vi "Main.vi"(10 "Sub Panel":refnum<vi>, 11 "Module Admin":refnum<class "Delacor_lib_QMH_Module Admin.lvclass">) -> ()   [LabVIEW 2020, in "Analisis.lvlib"]
doc: "This template is based off of the Queued Message Handler design pattern and the Queued Message Handler project template that ships with LabVIEW.\n\nThe main difference is that the queue is private to this module and communication between modules is performed via Broadcast and Request events.\n\nRequest events are wrapped in public API methods and are handled in the Event Handling Loop (EHL) of this VI. Any module can register for Broadcast events sent by this module. The EHL generates messages based on user interface actions.\n\nThe Message Handling Loop (MHL) processes messages generated by the EHL, or by other messages. The messages are string values, so new messages can be added easily to the Message Cases case structure in the MHL. Each message cluster can also provide an optional value for Message Data, which is a variant that can be converted to whatever message-specific data is required.\n_____\nBased on Delacor QMH Project Template 5.0.0.82."
uses:
  Analisis.lvlib
  <vilib>/Delacor/Delacor QMH/Libraries/Module Admin_class/Delacor_lib_QMH_Module Admin.lvclass
  Module Data--cluster.ctl
  <vilib>/vision/Image Controls.llb/IMAQ Image.ctl
  Stop Argument--cluster.ctl
  <vilib>/Delacor/Delacor QMH/Libraries/Message Queue_class/Delacor_lib_QMH_Message Queue.lvclass/Delacor_lib_QMH_Message Queue.ctl
  <vilib>/Delacor/Delacor QMH/Libraries/Module Admin_class/Delacor_lib_QMH_Module Admin.lvclass/Delacor_lib_QMH_Module Admin.ctl
  <vilib>/Delacor/Delacor QMH/Libraries/Message Queue_class/Delacor_lib_QMH_Enqueue Message (Single).vi
  <vilib>/Delacor/Delacor QMH/Libraries/Module Admin_class/Delacor_lib_QMH_Get External Launch.vi
  <vilib>/Utility/error.llb/Error Cluster From Error Code.vi
  <vilib>/ErrorRing/Error Ring.xnode
  <vilib>/Delacor/Delacor QMH/Libraries/Message Queue_class/Delacor_lib_QMH_Message Queue.lvclass
  Database/Database.lvlib
panel:
  out "Color:":string
  out "Image":T1(plugin-control)
  out "Codigo:":string
  out "Usuario:":string
  out "Letra:":string
  out "error out":errorcluster
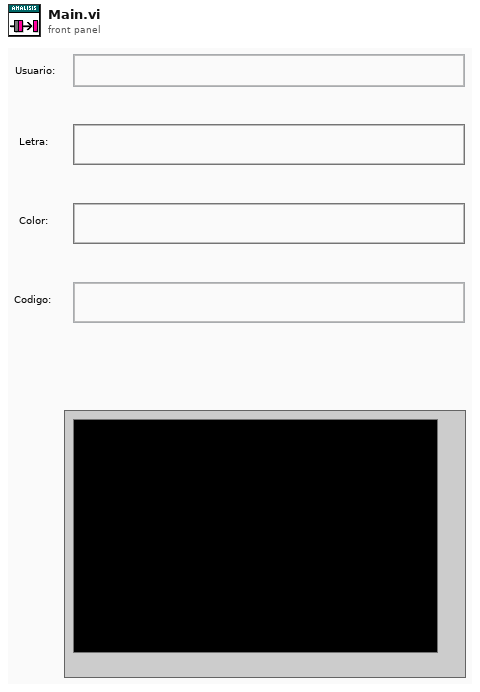
[diagram p1: front panel]
types:
  T1 = typedef "IMAQ Image.ctl" = refnum<image>
  T2 = typedef "Analisis.lvlib/Request Events--cluster.ctl" = cluster{"Stop Module":refnum<user-event>, "Show Panel":refnum<user-event>, "Hide Panel":refnum<user-event>, "Get Module Execution Status":refnum<user-event>, "Show Diagram":refnum<user-event>, "Start":refnum<user-event>, "stop analisis":refnum<user-event>}
  T3 = typedef "Analisis.lvlib/Module Data--cluster.ctl" = cluster{"Image Src":T1}
  T4 = enum32{"Invalid", "Standard", "Closed", "Hidden", "Minimized", "Maximized"}
  T5 = typedef "Analisis.lvlib/Stop Argument--cluster.ctl" = cluster{"Origin":string, "Exit via Stop Module Req?":bool, "Wait for Module to stop?":bool}
  T6 = enum32{"invalid lock state", "Not Locked", "Locked (No Password)", "Password-protected"}
  T7 = cluster{"Classes (Color Classification 1)[0]":string, "Classes (Color Classification 1)[1]":string, "Classes (Color Classification 1)[2]":string, "Classes (Color Classification 1)[3]":string, "Classes (Color Classification 1)[4]":string, "Classes (Color Classification 1)[5]":string, "Classes (Color Classification 1)[6]":string, "Classes (Color Classification 1)[7]":string, "Classes (Color Classification 1)[8]":string}
  T8 = cluster{"Complete Data (Barcode Reader 1)[0]":string, "Complete Data (Barcode Reader 1)[1]":string, "Complete Data (Barcode Reader 1)[2]":string, "Complete Data (Barcode Reader 1)[3]":string, "Complete Data (Barcode Reader 1)[4]":string, "Complete Data (Barcode Reader 1)[5]":string, "Complete Data (Barcode Reader 1)[6]":string, "Complete Data (Barcode Reader 1)[7]":string, "Complete Data (Barcode Reader 1)[8]":string}
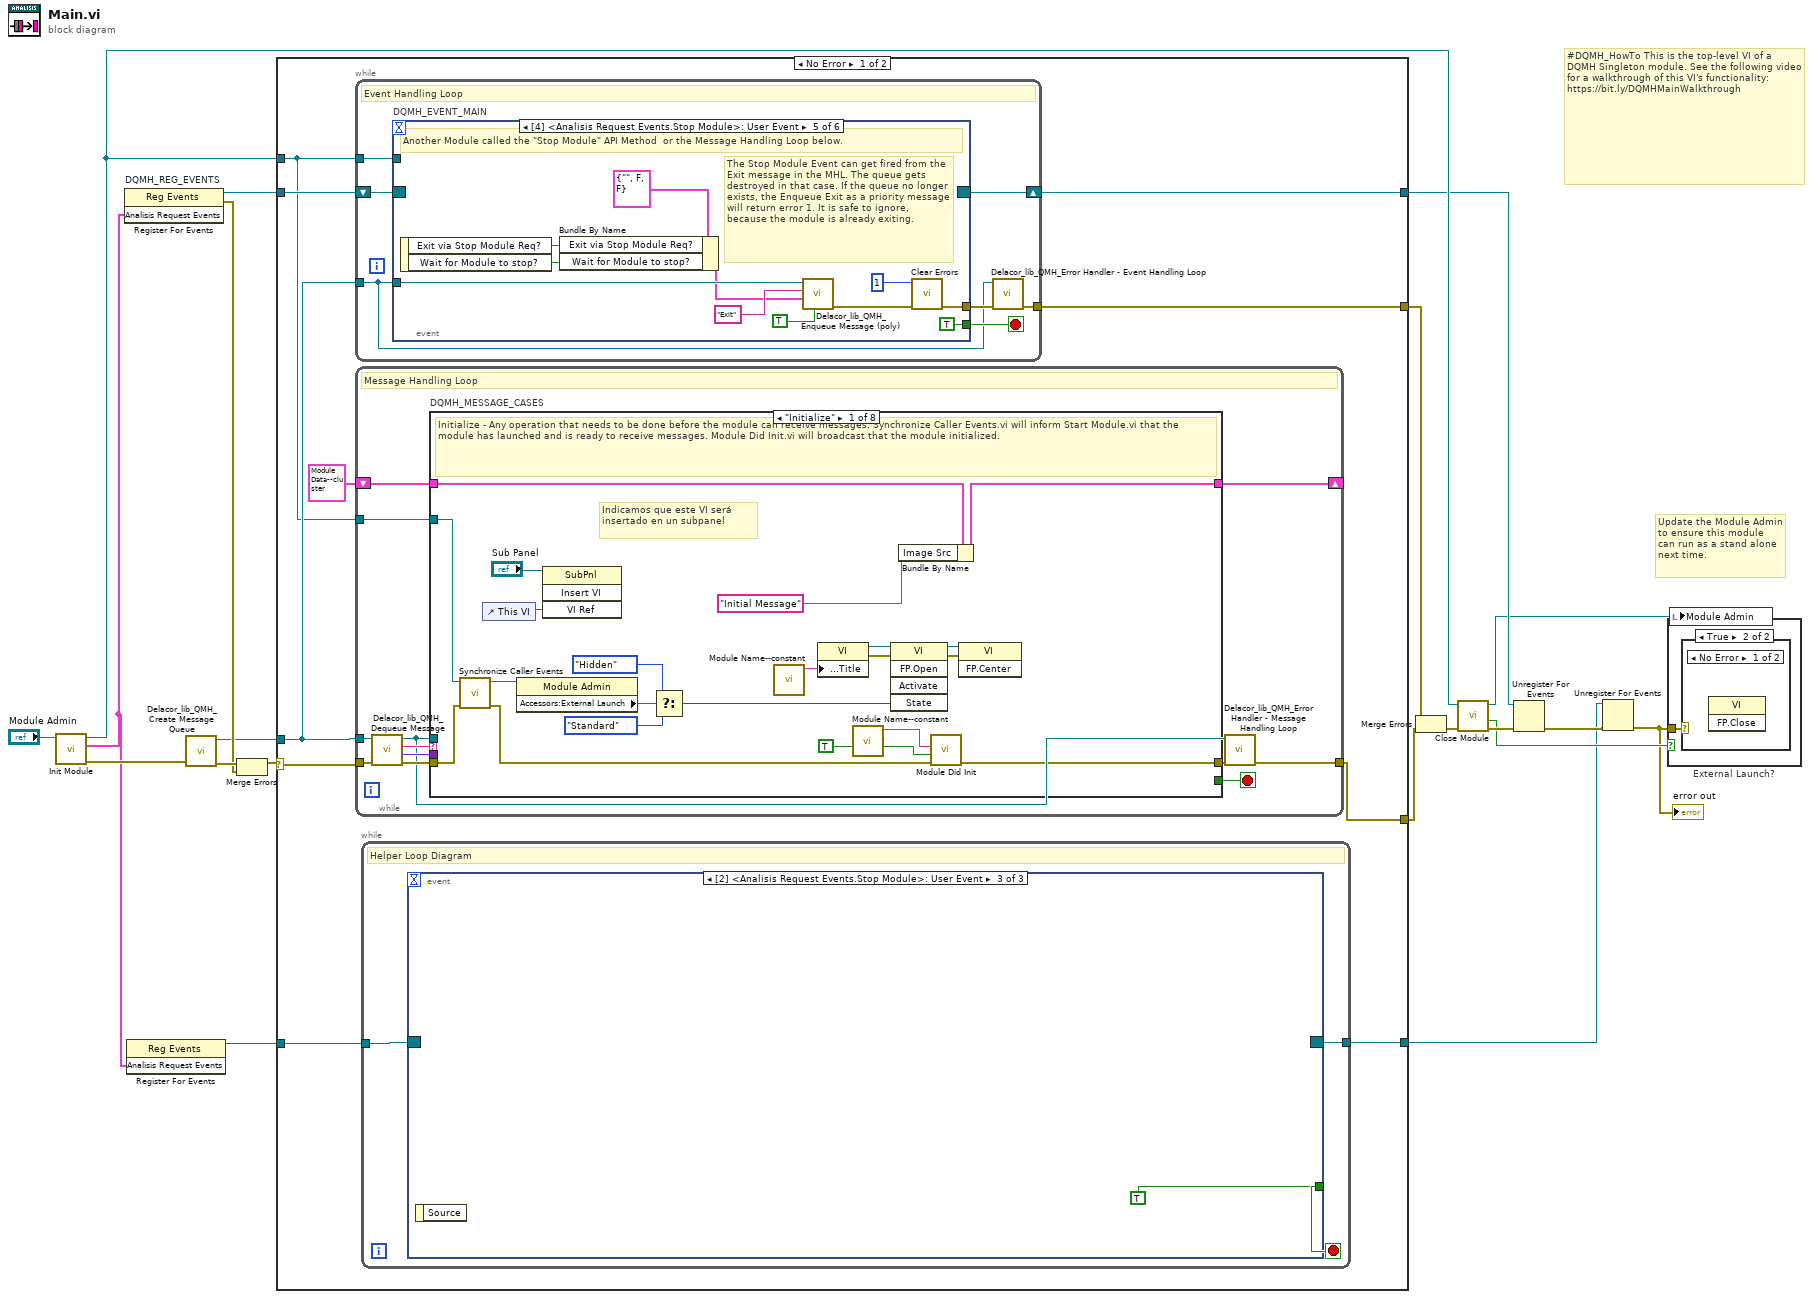
[diagram p0: block diagram]
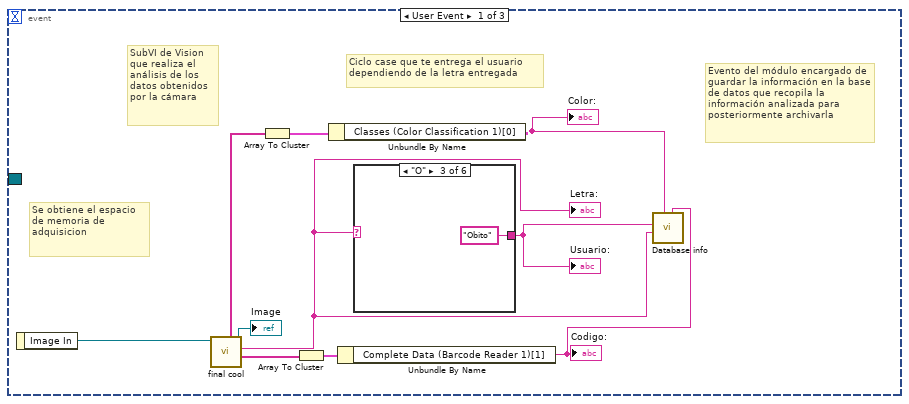
[diagram p2: hidden frame]
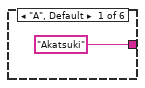
[diagram p3: hidden frame]
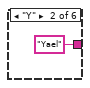
[diagram p4: hidden frame]
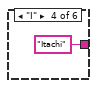
[diagram p5: hidden frame]
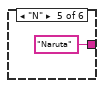
[diagram p6: hidden frame]
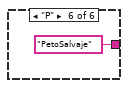
[diagram p7: hidden frame]
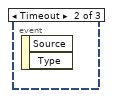
[diagram p8: hidden frame]
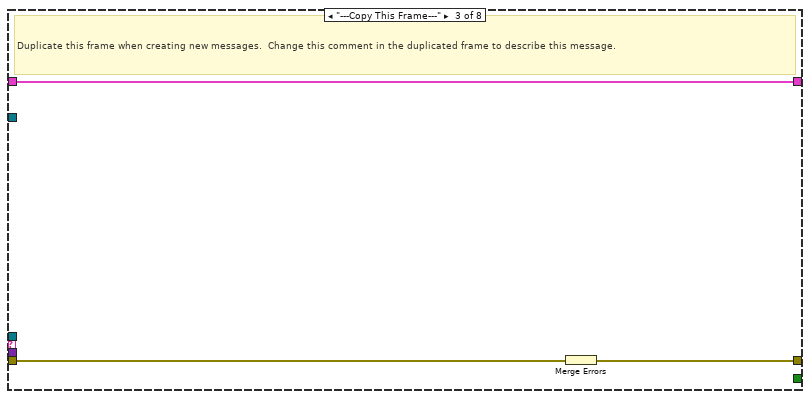
[diagram p10: hidden frame]
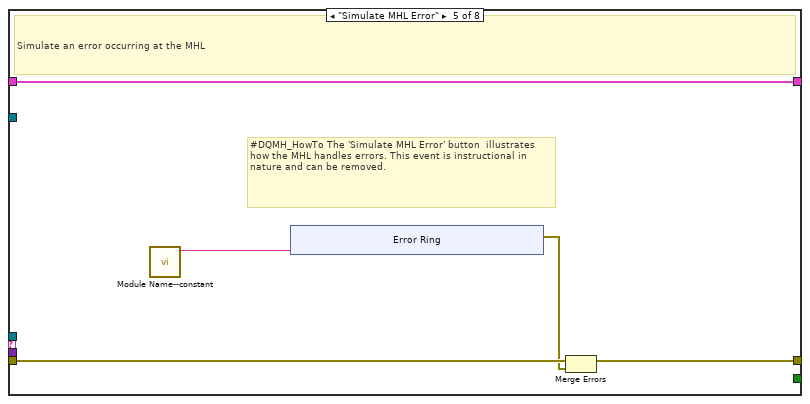
[diagram p12: hidden frame]
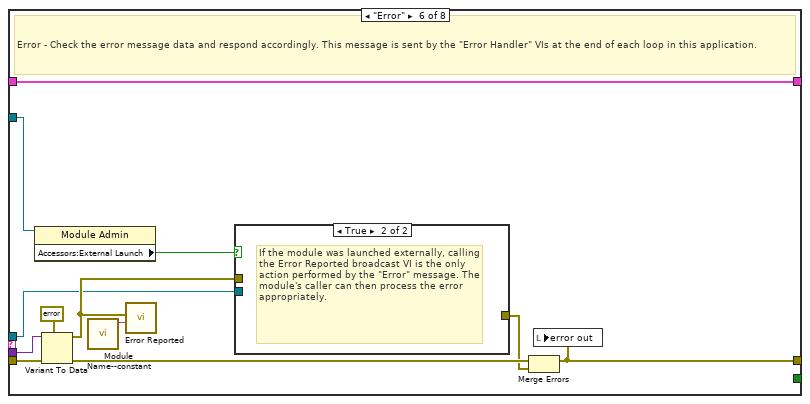
[diagram p13: hidden frame]
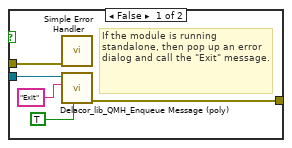
[diagram p14: hidden frame]
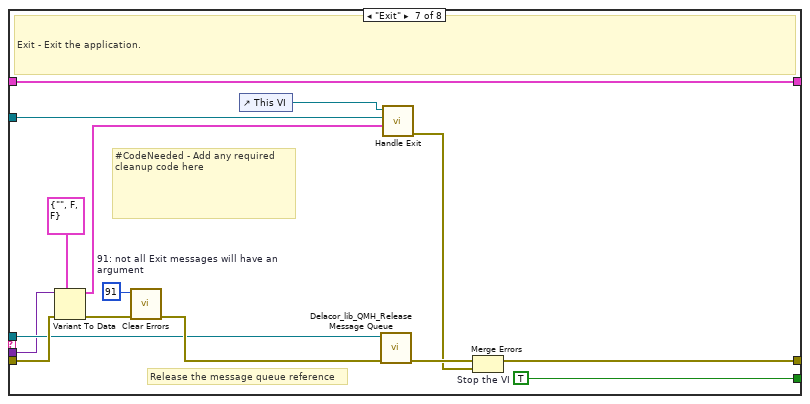
[diagram p15: hidden frame]
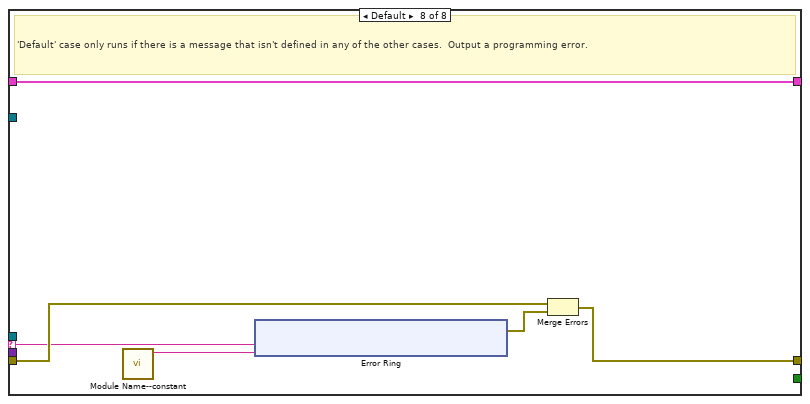
[diagram p16: hidden frame]
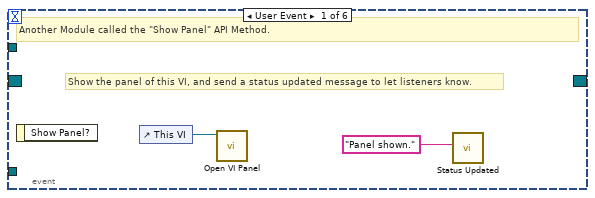
[diagram p17: hidden frame]
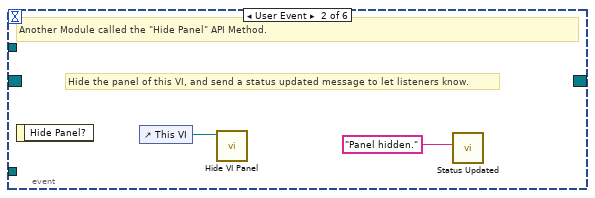
[diagram p18: hidden frame]
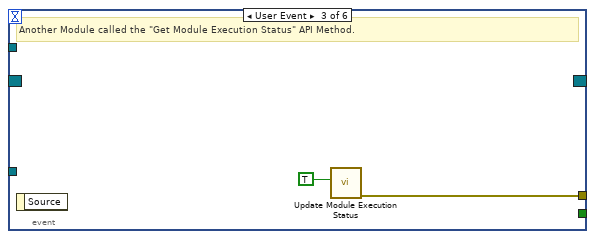
[diagram p19: hidden frame]
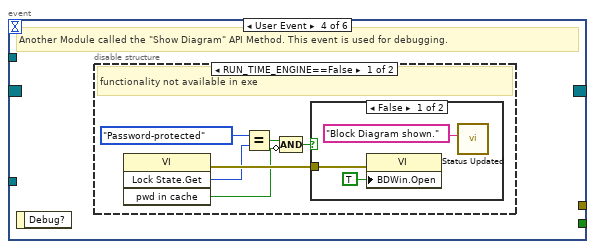
[diagram p20: hidden frame]
diagram:
  # "#DQMH_HowTo This is the top-level VI of a DQMH Singleton module. See the following video for a walkthrough of this VI's functionality: https://bit.ly/DQMHMainWalkthrough"
  # "Update the Module Admin to ensure this module can run as a stand alone next time."
  n1 = call "Init Module.vi"("Singleton Module Admin in"="Module Admin") -> ("error out"=w19:errorcluster, "Analisis Request Events"=w5:T2, "Singleton Module Admin out"=w12:refnum<class "Delacor_lib_QMH_Module Admin.lvclass">)  [unwired: 8 in]
  n2 = register-events "DQMH_REG_EVENTS"(w5) -> (reference out=w10:refnum<event-registration>, error out=w13:errorcluster)  [unwired: 2 in]
  n3 = register-events(w5) -> (reference out=w4:refnum<event-registration>)  [unwired: 2 in, 1 out]
  n4 = call <vilib>:"Delacor_lib_QMH_Create Message Queue.vi"("error in (no error)"=w19) -> ("error out"=w15:errorcluster, "Message Queue"=w9:refnum<class "Delacor_lib_QMH_Message Queue.lvclass">)  [unwired: 9 in]
  n5 = Merge Errors(w15, w13) -> (w14:errorcluster)
  n6 = case shown="No Error" w14 {
    selector: w14 -> [w28 w195]
    tunnel: [w30 w194] -> w20
    tunnel: [w27 w200] -> w11
    tunnel: w10 -> [w26 w200]
    tunnel: w9 -> [w25 w193]
    tunnel: [w29 _] -> w17
    tunnel: w12 -> [w24 w196]
    tunnel: w4 -> [w22 w192]
    tunnel: [w21 w192] -> w1
    frame No Error {
      n7 = while {
        tunnel: w25 -> [w149]
        shift-right: [w152] -> w27
        shift-left: w26 -> [w153]
        tunnel: [w154] -> w29
        tunnel: w24 -> [w150]
        stop <- w151 stop-if-true
        # "Event Handling Loop"
        n8 = event "DQMH_EVENT_MAIN" shown="[4] <Analisis Request Events.Stop Module>: User Event" {
          selector: w153 -> [_ _ _ _ _ _]
          dyn-events: [_ _ _ _ _ _] -> w152
          timeout: _ -> [_ _ _ _ _ _]
          tunnel: [_ _ _ _ TRUE ("Discard?") _] -> w151
          tunnel: w149 -> [_ _ _ _ w177 w184]
          tunnel: [_ _ w161 _ w180 w186] -> w155
          tunnel: w150 -> [_ _ _ _ _ w183]
          event User Event {
            # "Show the panel of this VI, and send a status updated message to let listeners know."
            # "Another Module called the \"Show Panel\" API Method."
            n9 = event-data() -> ()  [unwired: 1 in, 1 out]
            n10 = control-ref of="This VI"() -> (w157:refnum<vi>)
            n11 = call "Open VI Panel.vi"("VI"=w157) -> ()  [unwired: 10 in, 1 out]
            n12 = call "Status Updated.vi"("Status"="Panel shown." ("format string")) -> ()  [unwired: 10 in, 1 out]
          }
          event User Event {
            # "Hide the panel of this VI, and send a status updated message to let listeners know."
            # "Another Module called the \"Hide Panel\" API Method."
            n13 = event-data() -> ()  [unwired: 1 in, 1 out]
            n14 = control-ref of="This VI"() -> (w159:refnum<vi>)
            n15 = call "Hide VI Panel.vi"("VI"=w159) -> ()  [unwired: 10 in, 1 out]
            n16 = call "Status Updated.vi"("Status"="Panel hidden." ("format string")) -> ()  [unwired: 10 in, 1 out]
          }
          event User Event {
            # "Another Module called the \"Get Module Execution Status\" API Method."
            n17 = event-data() -> ()  [unwired: 1 in, 1 out]
            n18 = call "Update Module Execution Status.vi"("Running?"=TRUE) -> ("error out"=w161:errorcluster)  [unwired: 10 in]
          }
          event User Event {
            # "Another Module called the \"Show Diagram\" API Method. This event is used for debugging."
            n19 = event-data() -> ()  [unwired: 1 in, 1 out]
            n20 = disable-structure shown="RUN_TIME_ENGINE==False" {
              frame condition #0 (active) {
                # "functionality not available in exe"
                n21 = invoke class="VI" method="Lock State.Get"() -> (error out=w167:errorcluster, "Get Lock State"=w166:T6, "pwd in cache"=w163:bool)  [unwired: 4 in, 1 out]
                n22 = Equal?(x=T6."Password-protected", y=w166) -> (x = y?=w164:bool)
                n23 = Compound Arithmetic op=AND(w164, invert w163) -> (w162:bool)
                n24 = case shown="False" w162 {
                  tunnel: w167 -> [w170 _]
                  frame False {
                    n25 = property class="VI"(error in=w170, "BDWin.Open"=TRUE ("Block Diagram Window:Open")) -> ()  [unwired: 1 in, 2 out]
                    n26 = call "Status Updated.vi"("Status"="Block Diagram shown." ("format string")) -> ()  [unwired: 10 in, 1 out]
                  }
                  frame True {
                    # "Password-protected VI, and the password is not in the cache. Do not show the diagram."
                  }
                }
              }
              frame condition #1 {
              }
            }
          }
          event User Event {
            # "The Stop Module Event can get fired from the Exit message in the MHL. The queue gets destroyed in that case. If the queue no longer exists, the Enqueue Exit as a priority message will return error 1. It is safe to ignore, because the module is already exiting."
            # "Another Module called the \"Stop Module\" API Method  or the Message Handling Loop below."
            n27 = event-data() -> ("Exit via Stop Module Req?"=w173:bool, "Wait for Module to stop?"=w172:bool)  [unwired: 1 in]
            n28 = Bundle By Name(cluster=T5 {"Origin"="", "Exit via Stop Module Req?"=FALSE, "Wait for Module to stop?"=FALSE} ("Stop Argument"), "Exit via Stop Module Req?"=w173, "Wait for Module to stop?"=w172) -> (w171:T5)
            n29 = call-poly <vilib>:"Delacor_lib_QMH_Enqueue Message (poly).vi"("Priority Message? (F)"=TRUE, "Message Data"=w171, "Message"="Exit", "Message Queue in"=w177) -> ("error out"=w181:errorcluster)  [unwired: 6 in, 1 out]
            n30 = call <vilib>:"Clear Errors.vi"("error in (no error)"=w181, "specific error code to clear (0: all)"=1) -> ("error out"=w180:errorcluster)  [unwired: 4 in, 1 out]
          }
          event Panel Close? {
            w185 = TRUE  # Discard the event, the MHL is responsible for closing and stopping this VI.
            # "Hide the panel or send the 'Exit' message if the user clicks the 'X' on the module main VI panel."
            n31 = event-data() -> ()  [unwired: 1 in, 1 out]
            n32 = property class="Module Admin"(reference=w183) -> ("Accessors:External Launch"=w182:bool)  [unwired: 1 in, 2 out]
            n33 = case shown="True" w182 {
              tunnel: w184 -> [_ w190]
              tunnel: [_ w191] -> w186
              frame True {
                # "If externally launched, clicking the 'X' hides the panel, but doesn't close it."
                n34 = control-ref of="This VI"() -> (w187:refnum<vi>)
                n35 = call "Hide VI Panel.vi"("VI"=w187) -> ()  [unwired: 10 in, 1 out]
              }
              frame False {
                # "If run as a stand-alone VI, clicking the panel 'X' stops the VI."
                n36 = call-poly <vilib>:"Delacor_lib_QMH_Enqueue Message (poly).vi"("Priority Message? (F)"=TRUE, "Message"="Exit", "Message Queue in"=w190) -> ("error out"=w191:errorcluster)  [unwired: 7 in, 1 out]
              }
            }
            n37 = event-data("Discard?"=w185) -> ()  [unwired: 1 in, 1 out]
          }
        }
        n38 = call-dynamic "Delacor_lib_QMH_Error Handler - Event Handling Loop.vi"("error in (no error)"=w155, "Message Queue in"=w149) -> ("dup error in"=w154:errorcluster)  [unwired: 8 in, 1 out]
      }
      n39 = while {
        tunnel: w25 -> [w53]
        shift-right: [w57] -> _
        shift-left: T3 {"Image Src"=refnum} ("Data Cluster") -> [w58]
        tunnel: w28 -> [w61]
        tunnel: [w59] -> w30
        tunnel: w24 -> [w51]
        stop <- w56 stop-if-true
        # "Message Handling Loop"
        n40 = call-dynamic "Delacor_lib_QMH_Dequeue Message.vi"("error in (no error)"=w61, "Message Queue in"=w53) -> ("error out"=w60:errorcluster, "Message Data"=w54:variant, "Message"=w55:string, "Message Queue out"=w52:refnum<class "Delacor_lib_QMH_Message Queue.lvclass">)  [unwired: 6 in]
        n41 = case "DQMH_MESSAGE_CASES" shown="\"Initialize\"" w55 {
          selector: w55 -> [_ _ _ _ _ _ _ w136]
          tunnel: w52 -> [_ _ _ _ _ w106 w128 _]
          tunnel: w60 -> [w81 w85 w88 w90 w95 w113 w134 w138]
          tunnel: [w79 w85 w87 w90 w94 w109 w131 w139] -> w62
          tunnel: w58 -> [w70 w84 w86 w89 w92 w108 w127 w137]
          tunnel: [w69 w84 w86 w89 w92 w108 w127 w137] -> w57
          tunnel: [_ _ _ _ _ _ w126 _] -> w56
          tunnel: w54 -> [_ _ _ _ _ w107 w125 _]
          tunnel: w51 -> [w71 _ _ _ _ w105 w120 _]
          frame "Initialize" {
            # "Indicamos que este VI será insertado en un subpanel"
            # "Initialize - Any operation that needs to be done before the module can receive messages. Synchronize Caller Events.vi will inform Start Module.vi that the module has launched and is ready to receive messages. Module Did Init.vi will broadcast that the module initialized."
            n42 = call "Synchronize Caller Events.vi"("error in (no error)"=w81, "Singleton Module Admin in"=w71) -> ("error out"=w80:errorcluster, "Singleton Module Admin out"=w66:refnum<class "Delacor_lib_QMH_Module Admin.lvclass">)  [unwired: 8 in]
            n43 = control-ref of="This VI"() -> (w63:refnum<vi>)
            n44 = property class="Module Admin"(reference=w66) -> ("Accessors:External Launch"=w75:bool)  [unwired: 1 in, 2 out]
            n45 = invoke class="SubPnl" method="Insert VI"(reference="Sub Panel", "VI Ref"=w63) -> ()  [unwired: 2 in, 4 out]
            n46 = Select(t=T4."Hidden" ("State"), s=w75, f=T4."Standard" ("State")) -> (s? t:f=w72:T4)
            n47 = call "Module Name--constant.vi"() -> ("Module Name"=w78:string)  [unwired: 11 in]
            n48 = property class="VI"("Front Panel.Title"=w78) -> (reference out=w77:refnum<vi>, error out=w83:errorcluster)  [unwired: 2 in]
            n49 = call "Module Name--constant.vi"() -> ("Module Name"=w67:string)  [unwired: 11 in]
            n50 = invoke class="VI" method="FP.Open"(reference=w77, error in=w83, "State"=w72) -> (reference out=w76:refnum<vi>, error out=w82:errorcluster)  [unwired: 2 in, 3 out]
            n51 = Bundle By Name(cluster=w70, "Image Src"="Initial Message" ("Initial Message")) -> (w69:T3)
            n52 = call "Module Did Init.vi"("error in (no error)"=w80, "Initialized?"=TRUE, "Origin"=w67) -> ("error out"=w79:errorcluster)  [unwired: 8 in]
            n53 = invoke class="VI" method="FP.Center"(reference=w76, error in=w82) -> ()  [unwired: 1 in, 3 out]
          }
          frame "--- Module Specific ---" {
            # "Separator -- The following cases handle messages specific to this Module."
          }
          frame "---Copy This Frame---" {
            # "Duplicate this frame when creating new messages.  Change this comment in the duplicated frame to describe this message."
            n54 = Merge Errors(w88) -> (w87:errorcluster)
          }
          frame "--- Exit and Error Handling---" {
            # "Separator - The following cases handle errors and exit messages."
          }
          frame "Simulate MHL Error" {
            # "#DQMH_HowTo The 'Simulate MHL Error' button  illustrates how the MHL handles errors. This event is instructional in nature and can be removed."
            # "Simulate an error occurring at the MHL"
            n55 = call "Module Name--constant.vi"() -> ("Module Name"=w91:string)  [unwired: 11 in]
            n56 = xnode "Error Ring"("parameter 0"=w91) -> ("error out"=w93:errorcluster)
            n57 = Merge Errors(w95, w93) -> (w94:errorcluster)
          }
          frame "Error" {
            # "Error - Check the error message data and respond accordingly. This message is sent by the \"Error Handler\" VIs at the end of each loop in this application."
            n58 = property class="Module Admin"(reference=w105) -> ("Accessors:External Launch"=w104:bool)  [unwired: 1 in, 2 out]
            n59 = Variant To Data(error in=w113, type=errorcluster {"status"=FALSE, "code"=0, "source"=""} ("error constant"), Variant=w107) -> (data=w114:errorcluster, error out=w111:errorcluster)
            n60 = call "Module Name--constant.vi"() -> ("Module Name"=w103:string)  [unwired: 11 in]
            n61 = call "Error Reported.vi"("Additional Information"=w103, "Error"=w114) -> ()  [unwired: 9 in, 1 out]
            n62 = case shown="True" w104 {
              tunnel: [w119 _] -> w110
              tunnel: w106 -> [w117 _]
              tunnel: w114 -> [w118 _]
              frame False {
                # "If the module is running standalone, then pop up an error dialog and call the \"Exit\" message."
                n63 = call <vilib>:"Simple Error Handler.vi"("error in (no error)"=w118) -> ()  [unwired: 4 in, 5 out]
                n64 = call-poly <vilib>:"Delacor_lib_QMH_Enqueue Message (poly).vi"("Priority Message? (F)"=TRUE, "Message"="Exit", "Message Queue in"=w117) -> ("error out"=w119:errorcluster)  [unwired: 7 in, 1 out]
              }
              frame True {
                # "If the module was launched externally, calling the Error Reported broadcast VI is the only action performed by the \"Error\" message. The module's caller can then process the error appropriately."
              }
            }
            n65 = Merge Errors(w111, w110) -> (w109:errorcluster)
            n66 = local write "error out"(w109) -> ()
          }
          frame "Exit" {
            w124 = 91  # 91: not all Exit messages will have an argument
            w126 = TRUE  # Stop the VI
            # "Release the message queue reference"
            # "#CodeNeeded - Add any required cleanup code here"
            # "Exit - Exit the application."
            n67 = Variant To Data(error in=w134, type=T5 {"Origin"="", "Exit via Stop Module Req?"=FALSE, "Wait for Module to stop?"=FALSE} ("Stop Argument"), Variant=w125) -> (data=w122:T5, error out=w130:errorcluster)
            n68 = call <vilib>:"Clear Errors.vi"("error in (no error)"=w130, "specific error code to clear (0: all)"=w124) -> ("error out"=w133:errorcluster)  [unwired: 4 in, 1 out]
            n69 = control-ref of="This VI"() -> (w121:refnum<vi>)
            n70 = call-dynamic "Delacor_lib_QMH_Release Message Queue.vi"("error in (no error)"=w133, "Message Queue"=w128) -> ("error out"=w132:errorcluster)  [unwired: 9 in]
            n71 = call "Handle Exit.vi"("Stop Argument"=w122, "Admin in"=w120, "VI reference"=w121) -> ("error out"=w129:errorcluster)  [unwired: 7 in, 1 out]
            n72 = Merge Errors(w132, w129) -> (w131:errorcluster)
          }
          frame Default {
            # "'Default' case only runs if there is a message that isn't defined in any of the other cases.  Output a programming error."
            n73 = call "Module Name--constant.vi"() -> ("Module Name"=w135:string)  [unwired: 11 in]
            n74 = xnode "Error Ring"("parameter 0"=w136, "parameter 1"=w135) -> ("error out"=w140:errorcluster)
            n75 = Merge Errors(w138, w140) -> (w139:errorcluster)
          }
        }
        n76 = call-dynamic "Delacor_lib_QMH_Error Handler - Message Handling Loop.vi"("error in (no error)"=w62, "Message Queue in"=w52) -> ("dup error in"=w59:errorcluster)  [unwired: 8 in, 1 out]
      }
      n77 = while {
        tunnel: w22 -> [w33]
        tunnel: [w31] -> w21
        stop <- w32 stop-if-true
        # "Helper Loop Diagram"
        n78 = event shown="[2] <Analisis Request Events.Stop Module>: User Event" {
          selector: w33 -> [_ _ _]
          dyn-events: [_ _ _] -> w31
          timeout: _ -> [_ _ _]
          tunnel: [_ _ TRUE] -> w32
          event User Event {
            # "Ciclo case que te entrega el usuario dependiendo de la letra entregada"
            # "Evento del módulo encargado de guardar la información en la base de datos que recopila la información analizada para posteriormente archivarla"
            # "SubVI de Vision que realiza el análisis de los datos obtenidos por la cámara"
            # "Se obtiene el espacio de memoria de adquisicion"
            n79 = event-data() -> ("Image In"=w36:T1)  [unwired: 1 in]
            n80 = call "final cool.vi"("Image In"=w36) -> ("Complete Data (Barcode Reader 1)"=w38:string[], "String (OCR/OCV 1)"=w39:string, "Image Out"=→"Image":T1, "Classes (Color Classification 1)"=w40:string[])  [unwired: 6 in, 1 out]
            "Letra:" <- w39
            n81 = Array To Cluster(array=w40) -> (cluster=w42:T7)
            n82 = Array To Cluster(array=w38) -> (cluster=w37:T8)
            n83 = Unbundle By Name(w42) -> ("Classes (Color Classification 1)[0]"=w34:string)
            "Color:" <- w34
            n84 = Unbundle By Name(w37) -> ("Complete Data (Barcode Reader 1)[1]"=w35:string)
            "Codigo:" <- w35
            n85 = case shown="\"O\"" w39 {
              tunnel: ["Akatsuki" "Yael" "Obito" "Itachi" "Naruta" "PetoSalvaje"] -> w43
              frame "A", Default {
              }
              frame "Y" {
              }
              frame "O" {
              }
              frame "I" {
              }
              frame "N" {
              }
              frame "P" {
              }
            }
            "Usuario:" <- w43
            n86 = call "Database info.vi"("Codigo"=w35, "Color"=w34, "Letra"=w39, "usuario"=w43) -> ()  [unwired: 7 in, 1 out]
          }
          event Timeout {
            n87 = event-data() -> ()  [unwired: 1 in, 2 out]
          }
          event User Event {
            n88 = event-data() -> ()  [unwired: 1 in, 1 out]
          }
        }
      }
    }
    frame Error {
      # "Synchronize Caller Events.vi will inform Start Module.vi that the module has launched and will let the code calling Start Module.vi register for broadcasts and would permit the caller receive the broadcast that an error occurred at launch time."
      n89 = call-dynamic "Delacor_lib_QMH_Release Message Queue.vi"("error in (no error)"=w195, "Message Queue"=w193) -> ("error out"=w194:errorcluster)  [unwired: 9 in]
      n90 = call "Synchronize Caller Events.vi"("Singleton Module Admin in"=w196) -> ("error out"=w201:errorcluster)  [unwired: 9 in, 1 out]
      n91 = call "Module Name--constant.vi"() -> ("Module Name"=w199:string)  [unwired: 11 in]
      n92 = Format Into String(format string="An error occurred during initialization. %s is no longer running.", w199) -> (resulting string=w197:string)  [unwired: 2 in, 1 out]
      n93 = Merge Errors(w194, w201) -> (w202:errorcluster)
      n94 = call "Error Reported.vi"("Additional Information"=w197, "Error"=w202) -> ()  [unwired: 9 in, 1 out]
    }
  }
  n95 = Merge Errors(w17, w20) -> (w16:errorcluster)
  n96 = call "Close Module.vi"("error in (no error)"=w16, "Module Admin in"=w12) -> ("error out"=w18:errorcluster, "External Launch"=w6:bool, "Module Admin out"=w7:refnum<class "Delacor_lib_QMH_Module Admin.lvclass">)  [unwired: 7 in]
  n97 = Unregister For Events(event registration refnum=w11, error in=w18) -> (error out=w3:errorcluster)
  n98 = Unregister For Events(event registration refnum=w1, error in=w3) -> (error out=w2:errorcluster)
  "error out" <- w2
  n99 = case "External Launch?" shown="True" w6 {
    tunnel: w2 -> [_ w203]
    frame False {
    }
    frame True {
      n100 = case shown="No Error" w203 {
        frame No Error {
          n101 = invoke class="VI" method="FP.Close"() -> ()  [unwired: 3 in, 3 out]
        }
        frame Error {
          n102 = invoke class="VI" method="FP.Open"("Activate"=TRUE ("Activate?")) -> ()  [unwired: 4 in, 5 out]
        }
      }
    }
  }
  n103 = local write "Module Admin"(w7) -> ()
